vi "CAN-InsertFrame.vi"(6 "_FrameInfoIn":T2, 7 "ActIDs":sgl[](array[numeric])) -> (2 "_CANCELED":bool, 3 "_FrameInfo":T2)   [LabVIEW 2016]
uses:
  Shared/Typedefs/System-CAN-FrameInfo.ctl
  <vilib>/addons/Software Calibration Management/xSCM/Controls/ID and Element.ctl
  <vilib>/addons/Software Calibration Management/xSCM/SCM-API.lvlib
  Shared/DSI-Shared.lvlib
panel:
  in  "ID":T1
  in  "_CANCEL":bool
  in  "_OK":bool
  in  "_ExtID":bool caption="ID Length"
  in  "_Byte Order":u8(ring) caption="Byte Order" items=["Little Endian", "Big Endian"]
  in  "_Start Bit":u8 caption="Start Bit"
  in  "_Number of Bits":u8 caption="Number of Bits"
  out "_Units":string caption="Units"
  in  "_Identifier":u32 caption="Identifier" format="%.0x"
  out "_Name":string caption="Name (Right-Click to Modify)"
  in  "_Type":u16(ring) caption="Data Type" items=["Signed", "Unsigned", "IEEE Float"]
  in  "_Disable":bool
  in  "_Scaling Factor":sgl caption="Scaling Factor"
  in  "_Offset":sgl caption="Offset"
  in  "_Max":sgl caption="Max"
  in  "_Min":sgl caption="Min"
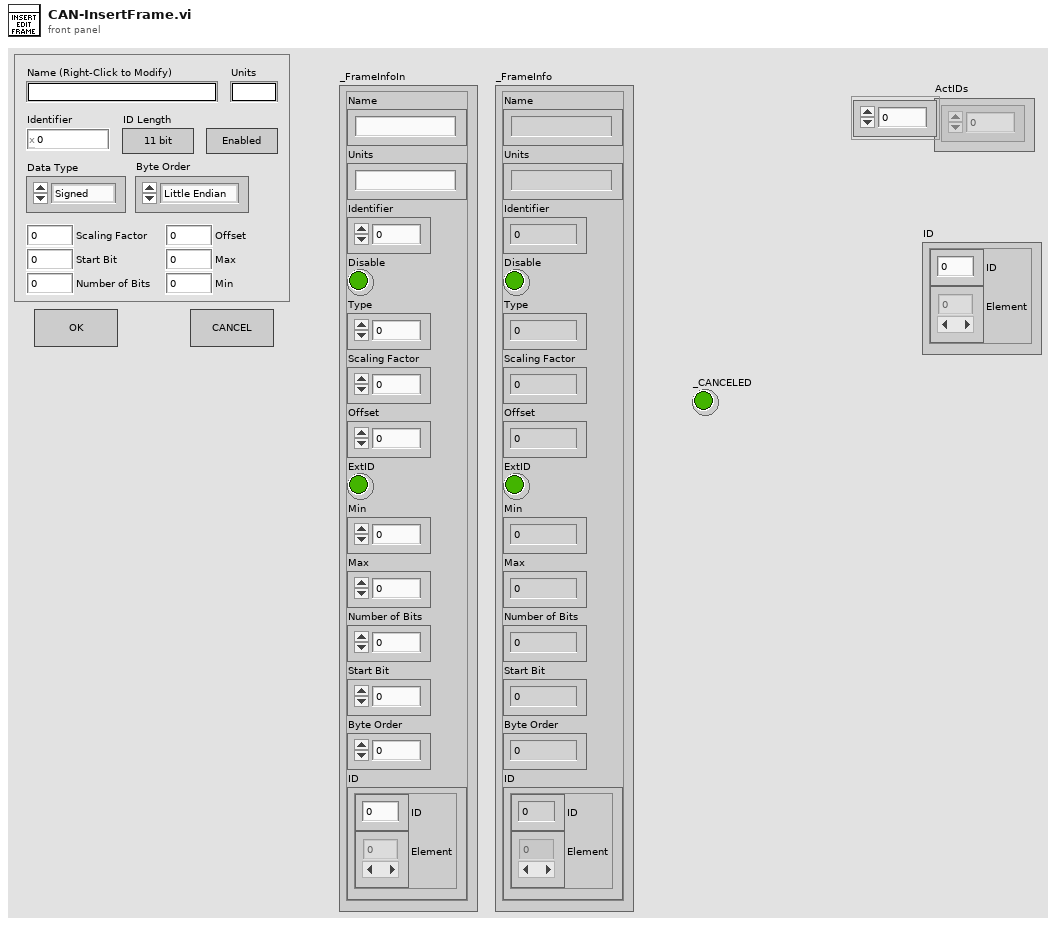
[diagram p1: front panel]
types:
  T1 = typedef "SCM-API.lvlib/ID and Element.ctl" = cluster{"ID":u32, "Element":i32[]}
  T2 = typedef "DSI-Shared.lvlib/System-CAN-FrameInfo.ctl" = cluster{"Name":string, "Units":string, "Identifier":u32, "Disable":bool, "Type":u8, "Scaling Factor":sgl, "Offset":sgl, "ExtID":bool, "Min":sgl, "Max":sgl, "Number of Bits":u8, "Start Bit":u8, "Byte Order":u8, "ID":T1}
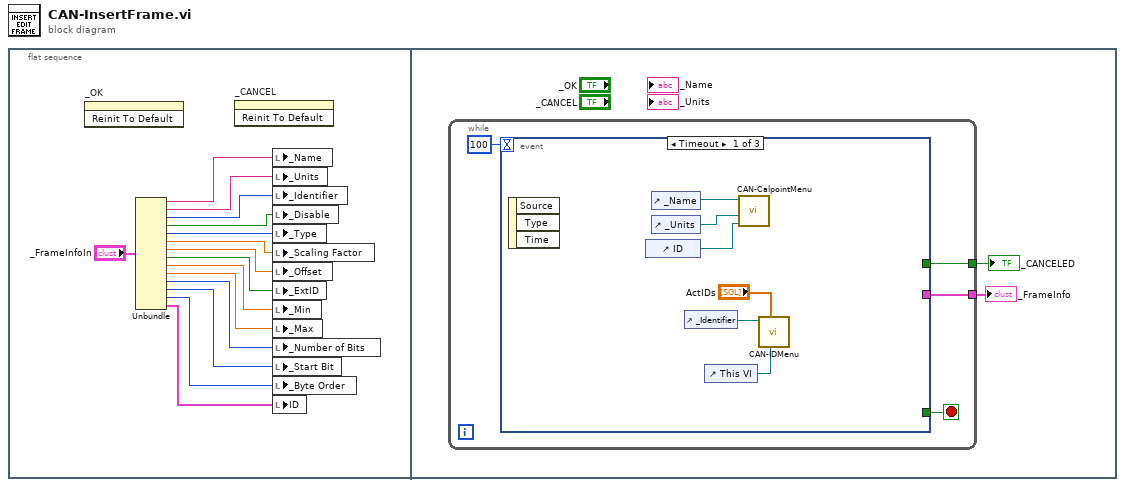
[diagram p0: block diagram]
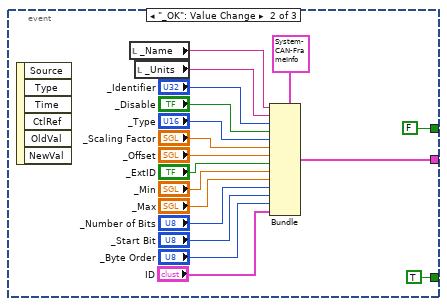
[diagram p2: hidden frame]
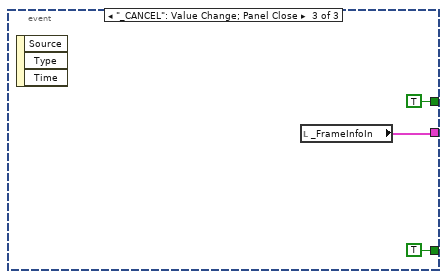
[diagram p3: hidden frame]
diagram:
  n1 = flat-sequence {
    frame #0 {
      n2 = invoke on="_OK" class="Bool (strict)" method="Reinit To Default"() -> ()  [unwired: 3 in, 3 out]
      n3 = Unbundle("_FrameInfoIn") -> ("Name"=w3:string, "Units"=w4:string, "Identifier"=w5:u32, "Disable"=w6:bool, "Type"=w7:u8, "Scaling Factor"=w8:sgl, "Offset"=w9:sgl, "ExtID"=w10:bool, "Min"=w11:sgl, "Max"=w12:sgl, "Number of Bits"=w13:u8, "Start Bit"=w14:u8, "Byte Order"=w15:u8, "ID"=w1:T1)
      n4 = invoke on="_CANCEL" class="Bool (strict)" method="Reinit To Default"() -> ()  [unwired: 3 in, 3 out]
      n5 = local write "_Name"(w3) -> ()
      n6 = local write "_Units"(w4) -> ()
      n7 = local write "_Identifier"(w5) -> ()
      n8 = local write "_Disable"(w6) -> ()
      n9 = local write "_Type"(w7) -> ()
      n10 = local write "_Scaling Factor"(w8) -> ()
      n11 = local write "_Offset"(w9) -> ()
      n12 = local write "_ExtID"(w10) -> ()
      n13 = local write "_Min"(w11) -> ()
      n14 = local write "_Max"(w12) -> ()
      n15 = local write "_Number of Bits"(w13) -> ()
      n16 = local write "_Start Bit"(w14) -> ()
      n17 = local write "_Byte Order"(w15) -> ()
      n18 = local write "ID"(w1) -> ()
    }
    frame #1 {
      n19 = while {
        tunnel: [w21] -> w16
        tunnel: [w19] -> w17
        stop <- w18 stop-if-true
        n20 = event shown="[0] Timeout" {
          selector: _ -> [_ _ _]
          dyn-events: _ -> [_ _ _]
          timeout: 100 -> [_ _ _]
          tunnel: [_ w42 w46] -> w21
          tunnel: [_ FALSE TRUE] -> w19
          tunnel: [_ TRUE TRUE] -> w18
          event Timeout {
            n21 = event-data() -> ()  [unwired: 1 in, 3 out]
            n22 = control-ref of="ID"() -> (w22:refnum<vi>)
            n23 = control-ref of="_Name"() -> (w27:refnum<vi>)
            n24 = control-ref of="_Units"() -> (w23:refnum<vi>)
            n25 = control-ref of="_Identifier"() -> (w24:refnum<vi>)
            n26 = control-ref of="This VI"() -> (w26:refnum<vi>)
            n27 = call "CAN-CalpointMenu.vi"("_ID"=w22, "_Unit"=w23, "_Name"=w27) -> ()  [unwired: 9 in]
            n28 = call "CAN-IDMenu.vi"("This VI"=w26, "ActIDs"="ActIDs", "_Identifier"=w24) -> ()  [unwired: 9 in]
          }
          event "_OK": Value Change {
            n29 = event-data() -> ()  [unwired: 1 in, 6 out]
            n30 = local read "_Name"() -> (w45:string)
            n31 = local read "_Units"() -> (w44:string)
            n32 = Bundle(cluster=T2 {"Name"="", "Units"="", "Identifier"=0, "Disable"=FALSE, "Type"=0, "Scaling Factor"=0.0, "Offset"=0.0, "ExtID"=FALSE, "Min"=0.0, "Max"=0.0, "Number of Bits"=0, "Start Bit"=0, "Byte Order"=0, "ID"={"ID"=0, "Element"=[]}} ("_FrameInfoIn"), "Name"=w45, "Units"=w44, "Identifier"="_Identifier", "Disable"="_Disable", "Type"="_Type", "Scaling Factor"="_Scaling Factor", "Offset"="_Offset", "ExtID"="_ExtID", "Min"="_Min", "Max"="_Max", "Number of Bits"="_Number of Bits", "Start Bit"="_Start Bit", "Byte Order"="_Byte Order", "ID"="ID") -> (w42:T2)
          }
          event "_CANCEL": Value Change; Panel Close {
            n33 = event-data() -> ()  [unwired: 1 in, 3 out]
            n34 = local read "_FrameInfoIn"() -> (w46:T2)
          }
        }
      }
      "_CANCELED" <- w17
      "_FrameInfo" <- w16
    }
  }
